vi "Apply Thrust.vi"(11 "Ship in":refnum<class "Ship.lvclass">) -> (3 "Ship out":refnum<class "Ship.lvclass">)   [LabVIEW 2015]
uses:
  Motion/Motion.lvclass
  Ship.lvclass
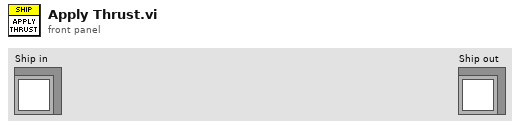
[diagram p1: front panel]
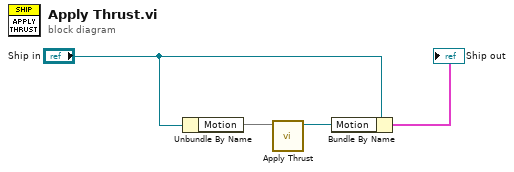
[diagram p0: block diagram]
diagram:
  n1 = Unbundle By Name("Ship in") -> ("Motion"=w4)
  n2 = call "Apply Thrust.vi"("Motion in"=w4) -> ("Motion out"=w1:refnum<class "Motion.lvclass">)  [unwired: 10 in]
  n3 = Bundle By Name(cluster="Ship in", "Motion"=w1) -> (→"Ship out":cluster{})
